vi "Get Supported SG Path Class Names.vi"(0 "SG Path PM Accessor in":refnum<class "SG Path PM Accessor Base.lvclass">, 11 "error in":errorcluster) -> (4 "SG Path PM Accessor out":refnum<class "SG Path PM Accessor Base.lvclass">, 6 "Supported SG Path Class Names":string[](array[string]), 15 "error out":errorcluster)   [LabVIEW 2023, in "RFFixtureCharact.Instruments.lvlib" / "SG Path PM Accessor Base.lvclass"]
uses:
  SG Path PM Accessor Base.lvclass
  RFPM/Scalar/Paths/SG Path/SG 18GHz Path.lvclass
  RMM/Scalar/Paths/SG 26GHz Path/SG 26GHz Path.lvclass
  RMM/Scalar/Paths/SG 54GHz Path/SG 54GHz Path.lvclass
  RMM/Scalar/Paths/SG 8GHz Path/SG 8GHz Path.lvclass
  PXI/Scalar/Paths/SG 8GHz Path/SG 8GHz Path.lvclass
  PXI/Scalar/Paths/SG 26GHz Path/SG 26GHz Path.lvclass
  SG Path PM Accessor Base.lvclass/SG Path PM Accessor Base.ctl
  D:/xixie/srd-semi-rfcal-software/AuxTools/STSRFFixtureCharactUtility/Source/Code Modules/Fixture/Public/Base Classes/Scalar/SG Abstract Path/SG Abstract Path.lvclass
  D:/xixie/srd-semi-rfcal-software/AuxTools/STSRFFixtureCharactUtility/Source/Code Modules/Fixture/Public/Base Classes/Scalar/Scalar Path/Scalar Path.lvclass
  D:/xixie/srd-semi-rfcal-software/AuxTools/STSRFFixtureCharactUtility/Source/Code Modules/Common/Base Classes/Path/Path.lvclass
  D:/xixie/srd-semi-rfcal-software/AuxTools/STSRFFixtureCharactUtility/Source/Code Modules/Fixture/RFPM/Scalar/Paths/SG Path/SG 18GHz Path.lvclass
  D:/xixie/srd-semi-rfcal-software/AuxTools/STSRFFixtureCharactUtility/Source/Code Modules/Fixture/RMM/Scalar/Paths/SG Path/SG Path.lvclass
  D:/xixie/srd-semi-rfcal-software/AuxTools/STSRFFixtureCharactUtility/Source/Code Modules/Fixture/Public/Base Classes/Scalar/SG Path/SG Path.lvclass
  D:/xixie/srd-semi-rfcal-software/AuxTools/STSRFFixtureCharactUtility/Source/Code Modules/Fixture/RMM/Scalar/Paths/SG 26GHz Path/SG 26GHz Path.lvclass
  D:/xixie/srd-semi-rfcal-software/AuxTools/STSRFFixtureCharactUtility/Source/Code Modules/Fixture/RMM/Scalar/Paths/SG 54GHz Path/SG 54GHz Path.lvclass
  D:/xixie/srd-semi-rfcal-software/AuxTools/STSRFFixtureCharactUtility/Source/Code Modules/Fixture/RMM/Scalar/Paths/SG 8GHz Path/SG 8GHz Path.lvclass
  D:/xixie/srd-semi-rfcal-software/AuxTools/STSRFFixtureCharactUtility/Source/Code Modules/Fixture/PXI/Scalar/Paths/SG 8GHz Path/SG 8GHz Path.lvclass
  D:/xixie/srd-semi-rfcal-software/AuxTools/STSRFFixtureCharactUtility/Source/Code Modules/Fixture/PXI/Scalar/Paths/SG 26GHz Path/SG 26GHz Path.lvclass
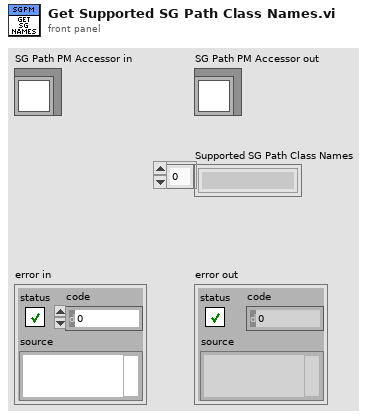
[diagram p1: front panel]
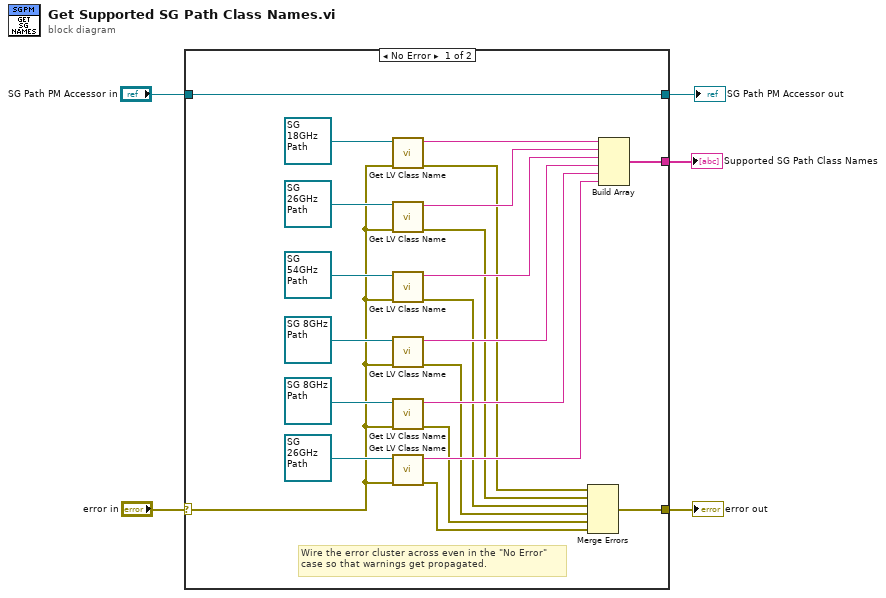
[diagram p0: block diagram]
diagram:
  n1 = case shown="No Error" "error in" {
    selector: "error in" -> [w12 w29]
    tunnel: [w13 w29] -> w4
    tunnel: [w27 w28] -> w2
    tunnel: "SG Path PM Accessor in" -> [w27 w28]
    tunnel: [w26 _] -> w1
    frame No Error {
      # "Wire the error cluster across even in the \"No Error\"\ncase so that warnings get propagated."
      n2 = call <vilib>:"Get LV Class Name.vi"("error in (no error)"=w12, "object"=refnum<class "SG 18GHz Path.lvclass"> refnum ("SG Path out")) -> ("error out"=w11:errorcluster, "class name"=w19:string)  [unwired: 8 in]
      n3 = call <vilib>:"Get LV Class Name.vi"("error in (no error)"=w12, "object"=refnum<class "SG 26GHz Path.lvclass"> refnum ("RFFixtureCharact.26GHz.lvlib:SG Path.lvclass")) -> ("error out"=w10:errorcluster, "class name"=w18:string)  [unwired: 8 in]
      n4 = call <vilib>:"Get LV Class Name.vi"("error in (no error)"=w12, "object"=refnum<class "SG 54GHz Path.lvclass"> refnum ("RFFixtureCharact.26GHz.lvlib:SG Path.lvclass")) -> ("error out"=w9:errorcluster, "class name"=w17:string)  [unwired: 8 in]
      n5 = call <vilib>:"Get LV Class Name.vi"("error in (no error)"=w12, "object"=refnum<class "SG 8GHz Path.lvclass"> refnum ("RFFixtureCharact.RMM.lvlib:SG 8GHz Path.lvclass")) -> ("error out"=w8:errorcluster, "class name"=w16:string)  [unwired: 8 in]
      n6 = call <vilib>:"Get LV Class Name.vi"("error in (no error)"=w12, "object"=refnum<class "SG 8GHz Path.lvclass"> refnum ("RFFixtureCharact.PXI.lvlib:SG 8GHz Path.lvclass")) -> ("error out"=w7:errorcluster, "class name"=w15:string)  [unwired: 8 in]
      n7 = call <vilib>:"Get LV Class Name.vi"("error in (no error)"=w12, "object"=refnum<class "SG 26GHz Path.lvclass"> refnum ("RFFixtureCharact.PXI.lvlib:SG 26GHz Path.lvclass")) -> ("error out"=w6:errorcluster, "class name"=w14:string)  [unwired: 8 in]
      n8 = Merge Errors(w11, w10, w9, w8, w7, w6) -> (w13:errorcluster)
      n9 = Build Array(w19, w18, w17, w16, w15, w14) -> (w26:string[])
    }
    frame Error {
    }
  }
  "error out" <- w4
  "SG Path PM Accessor out" <- w2
  "Supported SG Path Class Names" <- w1
